vi "Poll Robot and Accelerometer.vi"(8 "error in":errorcluster, 11 "UART in":refnum<visa-resource-name>) -> (0 "error out":errorcluster, 1 "Acceleration (g)":T4 {"z axis (g)" format="%.3f"; "y axis (g)" format="%.3f"; "x axis (g)" format="%.3f"}, 3 "UART out":refnum<visa-resource-name>, 4 "Kobuki Sensors  out":T1 {"Charger Source" items=["DISCHARGING"=0, "DOCKING_CHARGED"=2, "DOCKING_CHARGING"=6, "ADAPTER_CHARGED"=18, "ADAPTER_CHARGING"=22]}, 5 "net angle (deg)":i32, 7 "net distance (mm)":i32)   [LabVIEW 2016]
uses:
  shared/Accelerometer.ctl
  Kobuki/KobukiSensors.ctl
  Kobuki/Kobuki Bumps and WheelDrops.ctl
  Kobuki/Kobuki Buttons.ctl
panel:
  # "Electrical: charging, battery, OI mode"
  # "Sensors: bump, cliff, button, wheel drop"
  # "Motors:"
  # "Inertia"
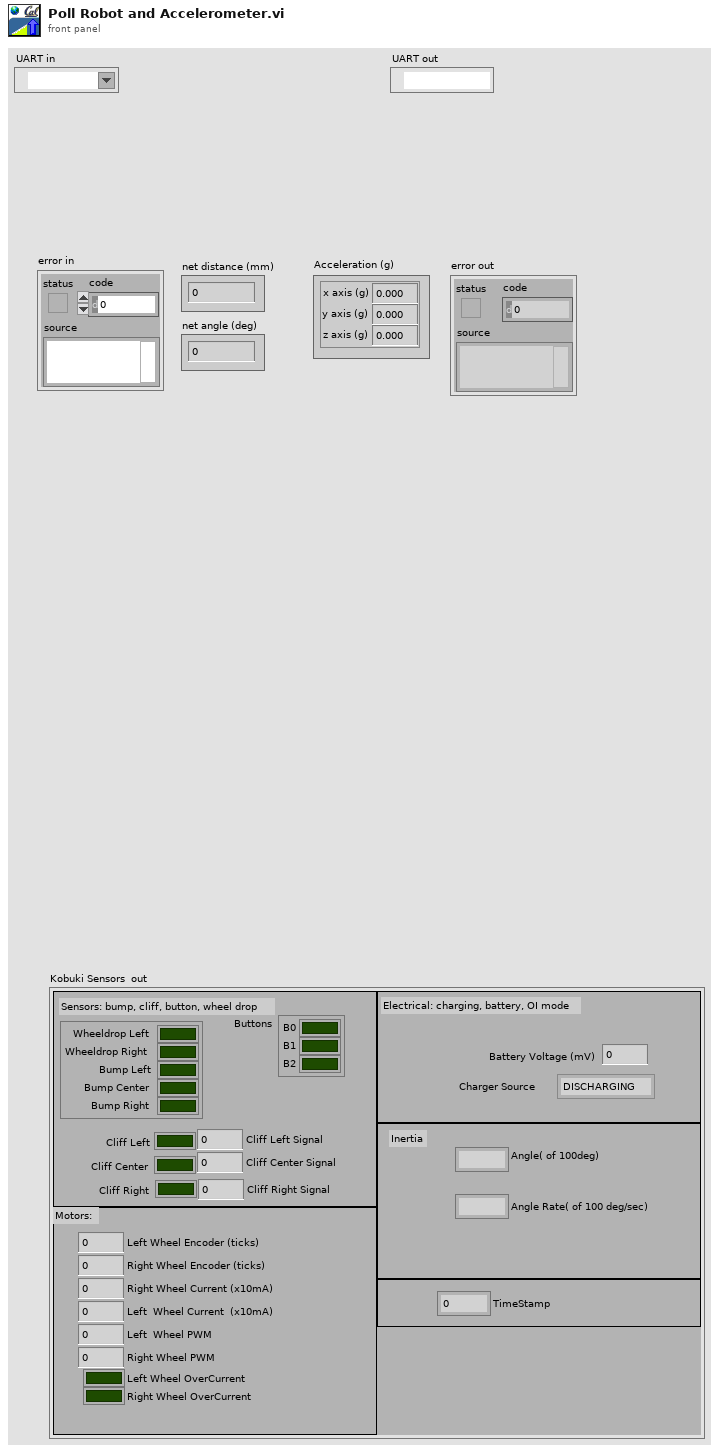
[diagram p1: front panel]
types:
  T1 = typedef "KobukiSensors.ctl" = cluster{"Bumps + Wheel Drops":T2, "Cliff Left":bool, "Cliff Center":bool, "Cliff Right":bool, "Cliff Left Signal":u16, "Cliff Center Signal":u16, "Cliff Right Signal":u16, "Buttons":T3, "Left Wheel Encoder (ticks)":u16, "Right Wheel Encoder (ticks) ":u16, "Left  Wheel PWM":i8, "Right Wheel PWM":i8, "Left Wheel OverCurrent":bool, "Right Wheel OverCurrent ":bool, "Right Wheel Current (x10mA)":i16, "Left  Wheel Current  (x10mA)":i16, "TimeStamp":u16, "Battery Voltage (mV)":i16, "Angle( of 100deg)":i16, "Angle Rate( of 100 deg/sec)":i16, "Charger Source ":i8}
  T2 = typedef "Kobuki Bumps and WheelDrops.ctl" = cluster{"Wheeldrop Left":bool, "Wheeldrop Right":bool, "Bump Left":bool, "Bump Center":bool, "Bump Right":bool}
  T3 = typedef "Kobuki Buttons.ctl" = cluster{"B0":bool, "B1":bool, "B2":bool}
  T4 = typedef "Accelerometer.ctl" = cluster{"x axis (g)":dbl, "y axis (g)":dbl, "z axis (g)":dbl}
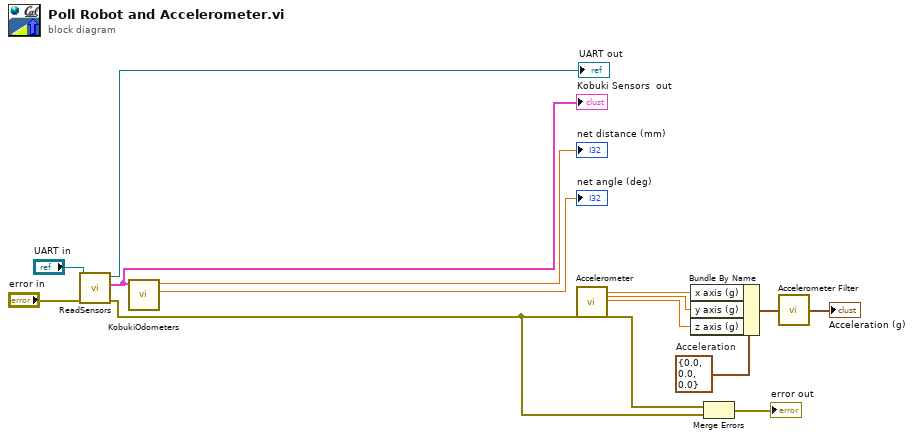
[diagram p0: block diagram]
diagram:
  w13 = T4 {"x axis (g)"=0.0, "y axis (g)"=0.0, "z axis (g)"=0.0}  # Acceleration
  n1 = call "ReadSensors.vi"("error in"="error in", "UART in"="UART in") -> ("error out"=w2:errorcluster, "Kobuki Sensors  out"=w5:T1, "UART out"=→"UART out":refnum<visa-resource-name>)  [unwired: 7 in]
  "Kobuki Sensors  out" <- w5
  n2 = call "KobukiOdometers.vi"("Kobuki Sensors  in"=w5) -> ("NetAngle"=→"net angle (deg)":dbl, "NetDistance"=→"net distance (mm)":dbl)  [unwired: 7 in, 2 out]
  n3 = call "Accelerometer"("error in (no error)"=w2) -> ("X-Axis"=w12:dbl, "Y-Axis"=w11:dbl, "Z-Axis"=w10:dbl, "error out"=w1:errorcluster)  [unwired: 23 in]
  n4 = Bundle By Name(cluster=w13, "x axis (g)"=w12, "y axis (g)"=w11, "z axis (g)"=w10) -> (w9:T4)
  n5 = Merge Errors(w1, w2) -> (→"error out":errorcluster)
  n6 = call "Accelerometer Filter.vi"("accelerometer (g)"=w9) -> ("filtered accelerometer (g)"=→"Acceleration (g)":T4)  [unwired: 3 in]
